vi "Main Loop.vi"(8 "error in (no error)":errorcluster, 10 "Chart Notifier":refnum<notifier>, 11 "Message Queues":T1) -> (0 "error out":errorcluster)   [LabVIEW 2018, in "Flow Module.lvlib" / "Flow Module Engine.lvlib"]
uses:
  Flow Module Engine.lvlib
  Flow Message Queues.ctl
  support/Message Queue/Message Cluster.ctl
  State Cluster.ctl
  State Enum.ctl
  Feed Module/Controls/Flow Module Settings Cluster.ctl
  Bronkhorst M13 Flow Meter/Settings Cluster.ctl
  Bronkhorst M14 Flow Meter/Settings Cluster.ctl
  Feed Module/Controls/Flow Module Display.ctl
  <vilib>/Platform/TimedLoop/XDataNode/timing_clust.ctl
  <vilib>/Platform/TimedLoop/XDataNode/nitl_modes.ctl
  <vilib>/Platform/TimedLoop/XDataNode/wakeup.ctl
  Tag VIs/Tag FGV Operation Enum.ctl
  support/Message Queue/Enqueue Message (Single).vi
  <vilib>/Platform/TimedLoop/XDataNode/XDataNode.xnode
  support/Message Queue/Message Queue.lvlib
  <vilib>/Platform/TimedLoop/XDataNode/XDNodeRunTimeDep.lvlib
  Flow Module.lvlib
  Shared Variables/Dynamic Shared Variables.lvlib
  support/Support Library.lvlib
  Bronkhorst M14 Flow Meter/Bronkhorst M14 Flow Meter.lvlib
  Bronkhorst M13 Flow Meter/Bronkhorst M13 Flow Meter.lvlib
panel:
  out "Period (s)":dbl format="%_4g"
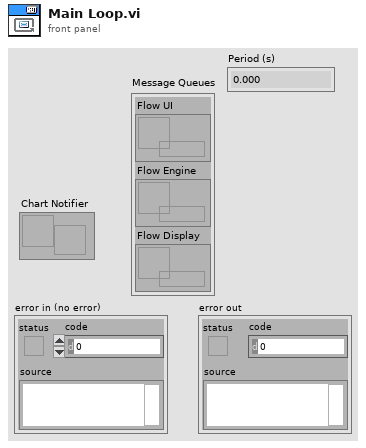
[diagram p1: front panel]
types:
  T1 = typedef "Flow Module.lvlib/Flow Message Queues.ctl" = cluster{"Flow UI":refnum<queue>, "Flow Engine":refnum<queue>, "Flow Display":refnum<queue>}
  T2 = typedef "Flow Module.lvlib/Flow Module Engine.lvlib/State Cluster.ctl" = cluster{"State":T3, "Start Time":timestamp, "Configuration":T4, "Current Time":timestamp, "First Iteration":bool, "Data":cluster{"Flow Meter Read(g/min)":dbl, "Density":dbl, "Temp (C)":dbl, "Totalized":dbl}, "Process Name":string, "Log Started":bool}
  T3 = typedef "Flow Module.lvlib/Flow Module Engine.lvlib/State Enum.ctl" = enum16{"Measuring", "Idle"}
  T4 = typedef "Flow Module.lvlib/Flow Module Settings Cluster.ctl" = cluster{"Cycle Period":dbl, "Flow Meter Type":string, "Bronkhorst M13 Settings":T5, "Bronkhorst M14 Settings":T6, "Reset Totalizer":bool}
  T5 = typedef "Bronkhorst M13 Flow Meter.lvlib/Settings Cluster.ctl" = cluster{"VISA resource name":refnum<visa-resource-name>, "Simulated?":bool, "Smoothing Steps":i32}
  T6 = typedef "Bronkhorst M14 Flow Meter.lvlib/Settings Cluster.ctl" = cluster{"VISA resource name":refnum<visa-resource-name>, "Simulated?":bool, "Smoothing Steps":i32}
  T7 = typedef "XDNodeRunTimeDep.lvlib/timing_clust.ctl" = cluster{"Expected End [f-1]":u64, "Actual End [f-1]":u64, "Finished Late? [f-1]":bool, "Expected End [i-1]":u64, "Actual End [i-1]":u64, "Finished Late? [i-1]":bool, "Expected Start [i]":u64, "Actual Start [i]":u64, "Expected Start [f]":u64, "Actual Start [f]":u64, "Source Name":string, "Structure Name":string, "Period":i64, "Deadline":i64, "Offset":i64, "Start":i64, "Priority":i32, "Timeout":i32, "Mode":T8, "Wakeup Reason":T9, "Error":errorcluster, "Source Type":string, "Secondary Source Type":string, "Global End Time":u64, "Global Start Time":u64, "Frame Duration":u64, "Iteration Duration":u64, "Assigned CPU":i32, "I/O Scan Engine Mode":u32}
  T8 = typedef "XDNodeRunTimeDep.lvlib/nitl_modes.ctl" = enum32{"No Change", "Process missed periods, maintain original phase", "Discard missed periods, maintain original phase", "Process missed periods, ignore original phase", "Discard missed periods, ignore original phase"}
  T9 = typedef "XDNodeRunTimeDep.lvlib/wakeup.ctl" = enum32{"Normal", "Aborted", "Asynchronous wakeup", "Timing source error", "Timed loop error", "Timeout"}
  T10 = cluster{"enable? (F)":bool, "name":string, "alarm on":bool, "priority":u32, "ack type":enum16{"Auto", "User", "None", "Each Occurrence"}, "area":string, "description":string, "log? (T)":bool}
  T11 = typedef "Tag FGV Operation Enum.ctl" = enum16{"Init", "Set Notification Queue", "Create Tag", "Commit", "Write Tag (Numeric)", "Write Tag (Boolean)", "Read All Tags", "Read One Tag", "Delete Tag Category", "Set Alarm Parameters (Numeric)", "Set Alarm Parameters (Boolean)", "Enable All Alarms", "Disable All Alarms", "Delete All Tags", "Read Alarms", "Ack Alarm", "Read Alarm Parameters (Numeric)", "Read Alarm Parameters (Boolean)"}
  T12 = enum32{"u32BitField", "bool", "double", "string", "int8", "uint8", "int16", "uint16", "int32", "uint32", "int64", "uint64", "single", "double waveform", "int16 waveform", "array of boolean", "array of int8", "array of uint8", "array of int16", "array of uint16", "array of int32", "array of uint32", "array of int64", "array of uint64", "array of single", "array of double", "array of double waveform", "array of int16 waveform", "array of string", "variant", "timestamp", "fixed point", "custom"}
  T13 = typedef "Flow Module.lvlib/Flow Module Display.ctl" = cluster{"Flow Value":dbl, "Cycle Period":dbl, "Density":dbl, "Temp":dbl, "Totalized":dbl}
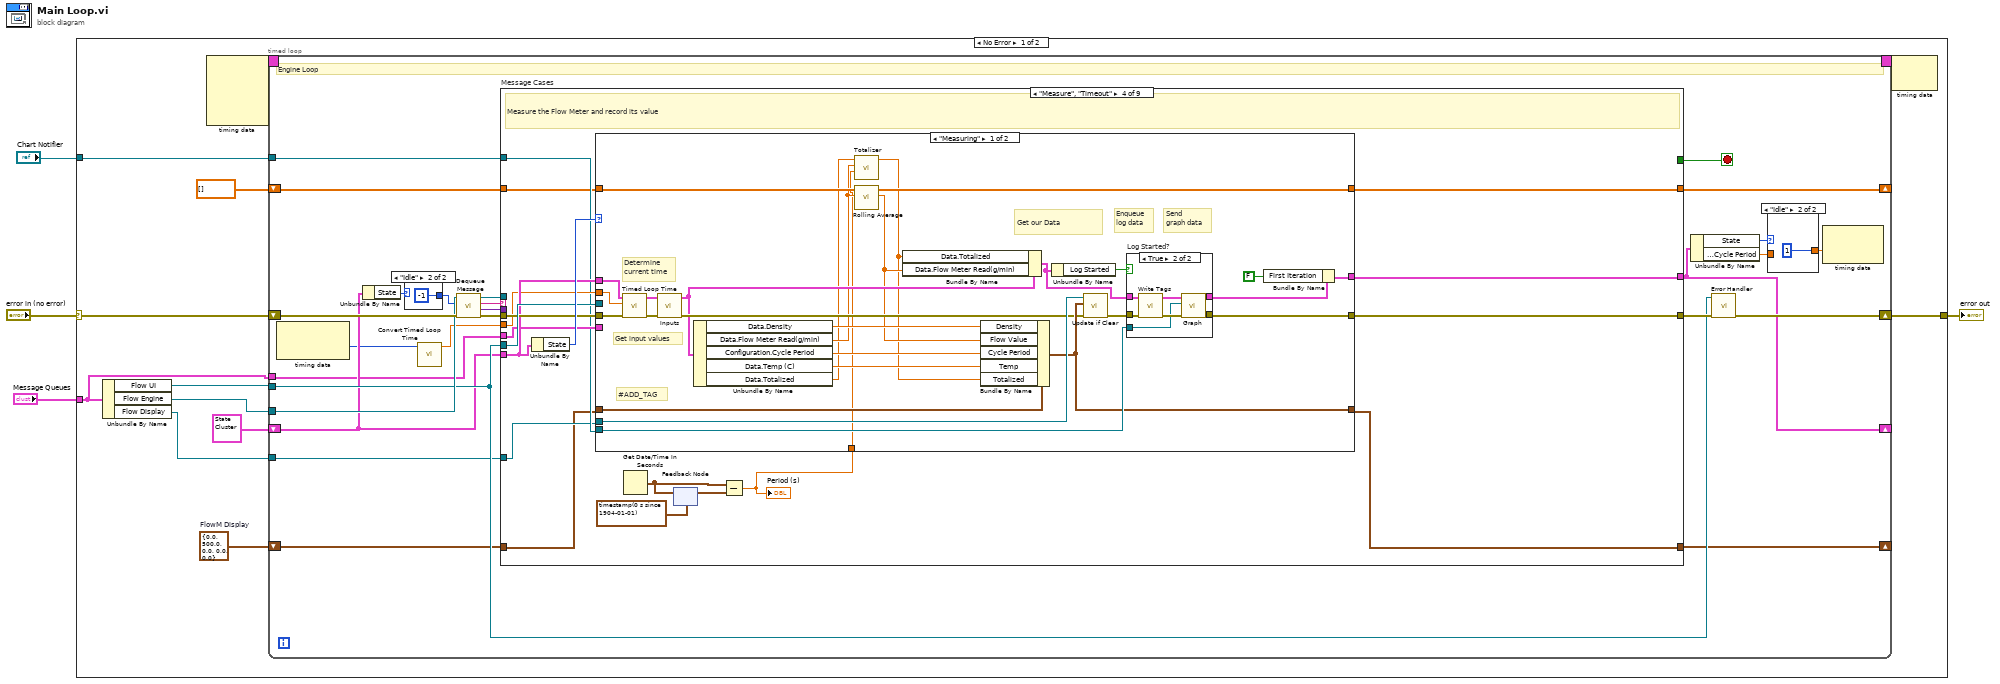
[diagram p0: block diagram]
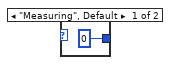
[diagram p3: hidden frame]
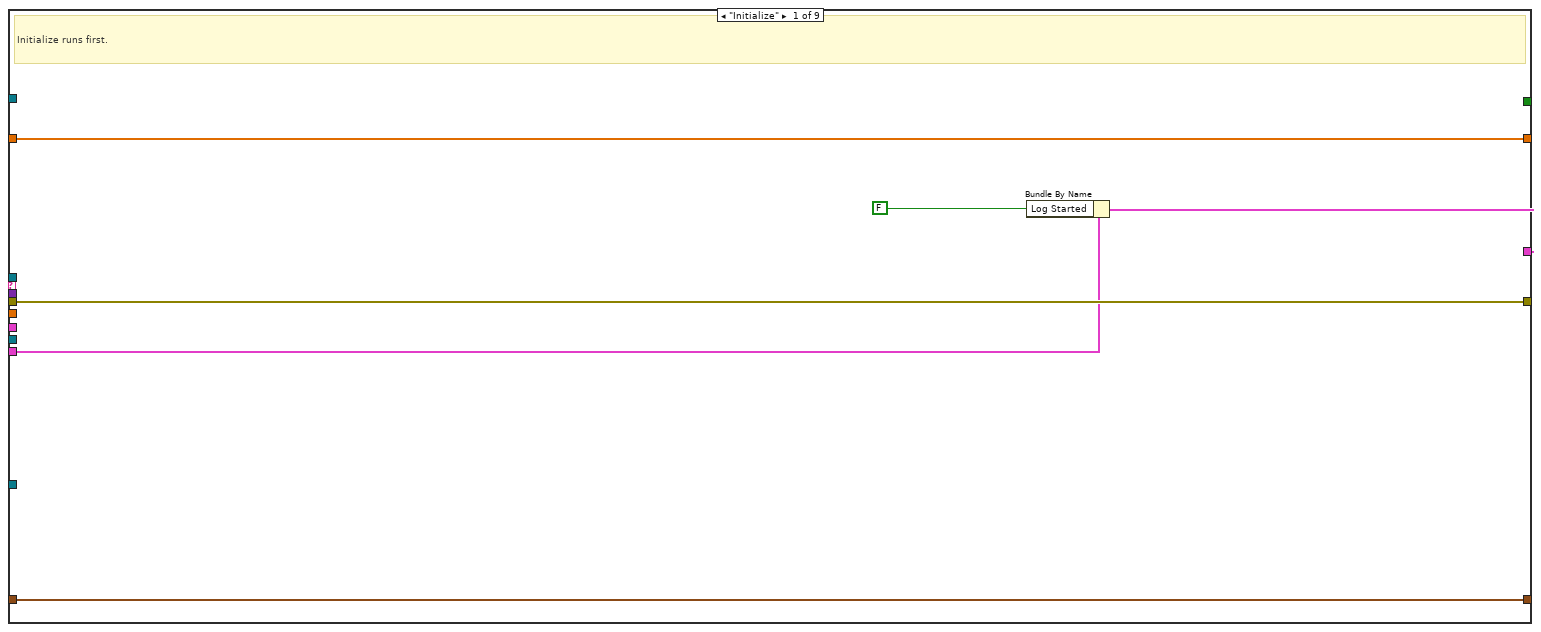
[diagram p4: hidden frame]
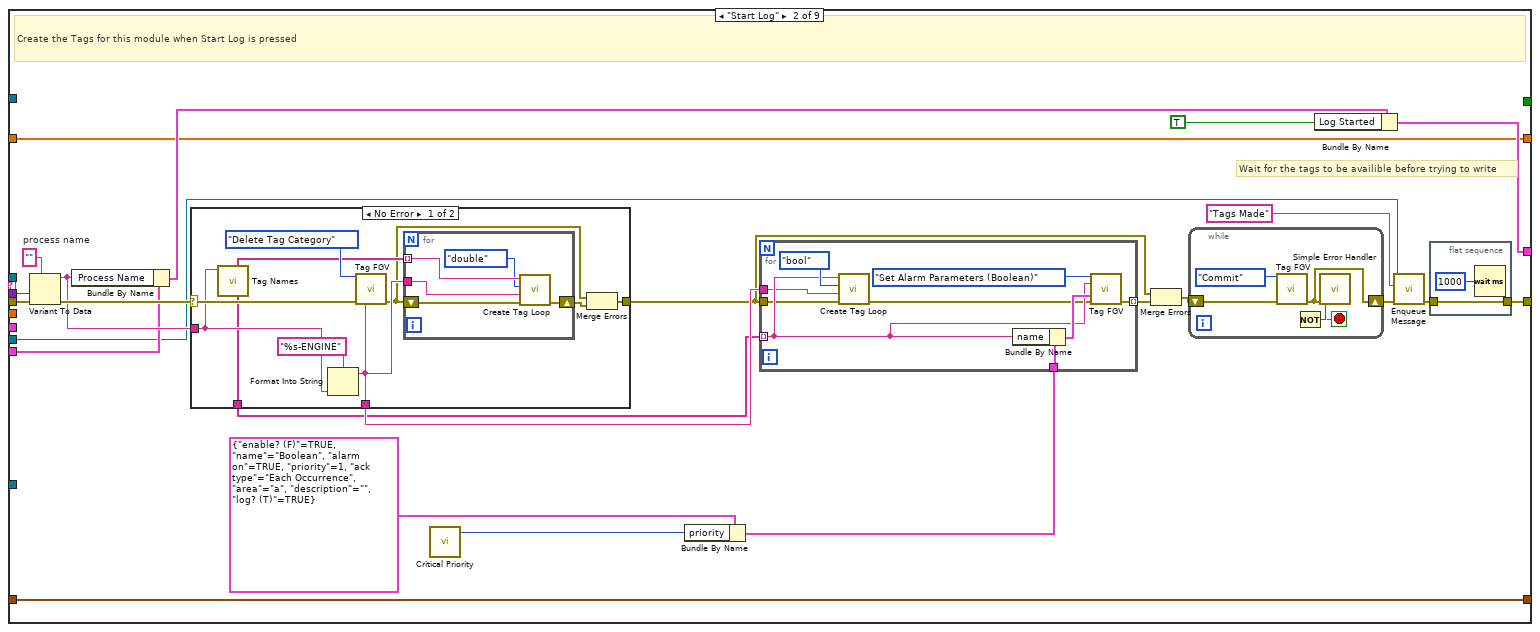
[diagram p5: hidden frame]
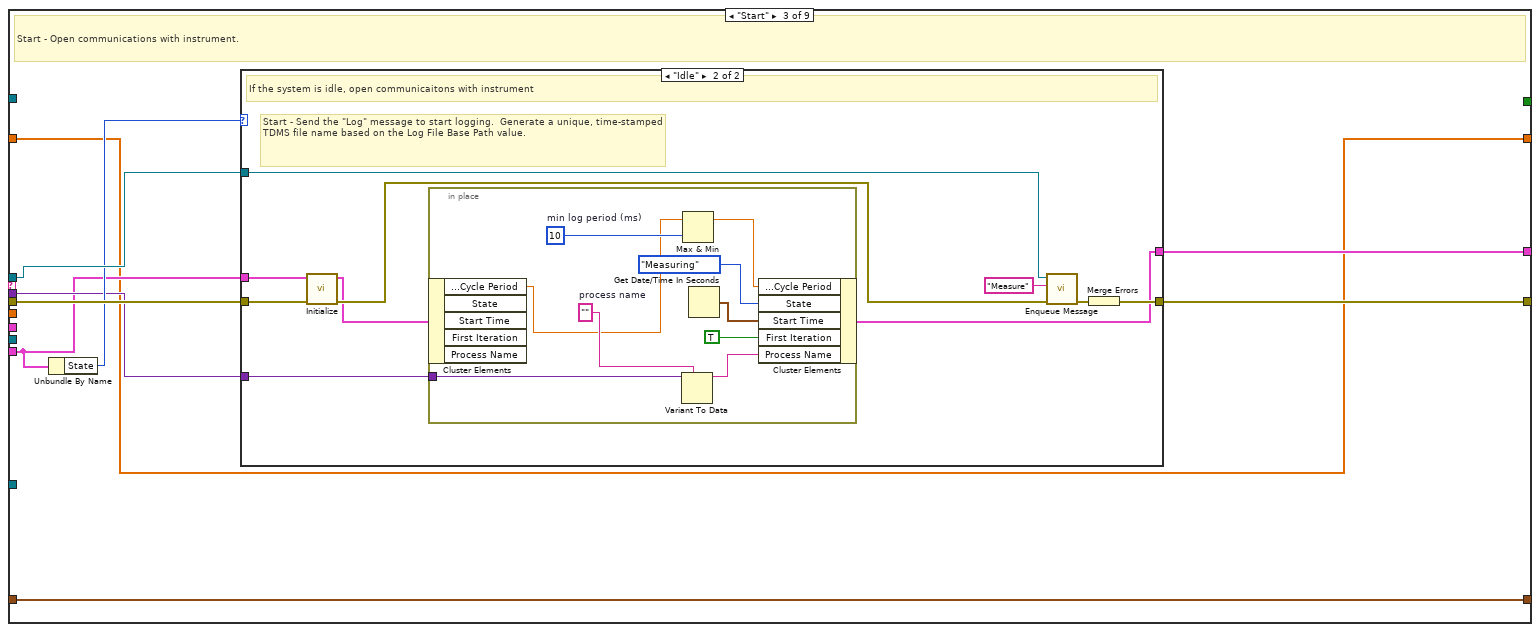
[diagram p7: hidden frame]
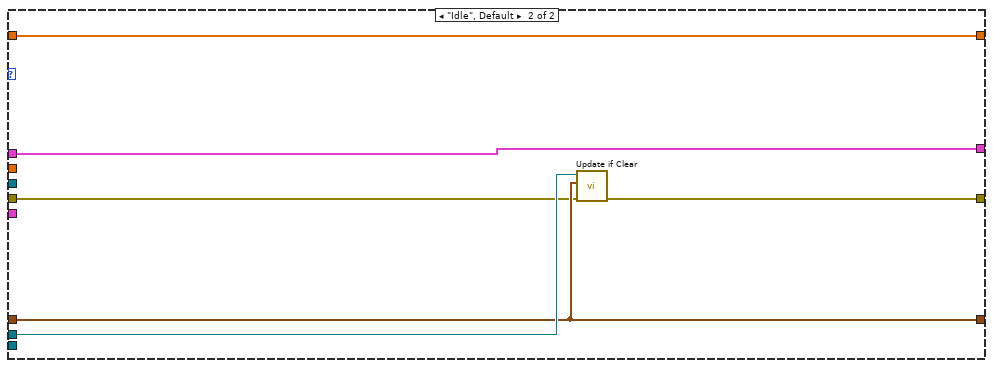
[diagram p10: hidden frame]
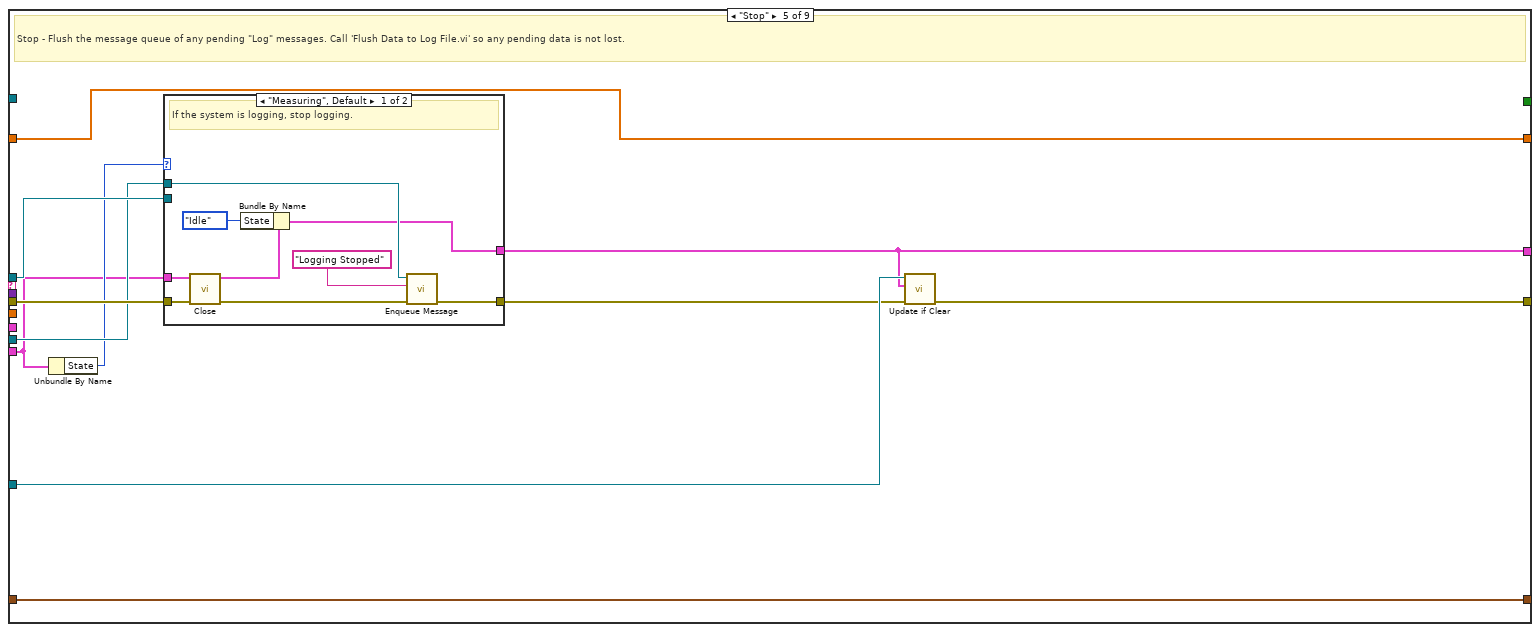
[diagram p11: hidden frame]
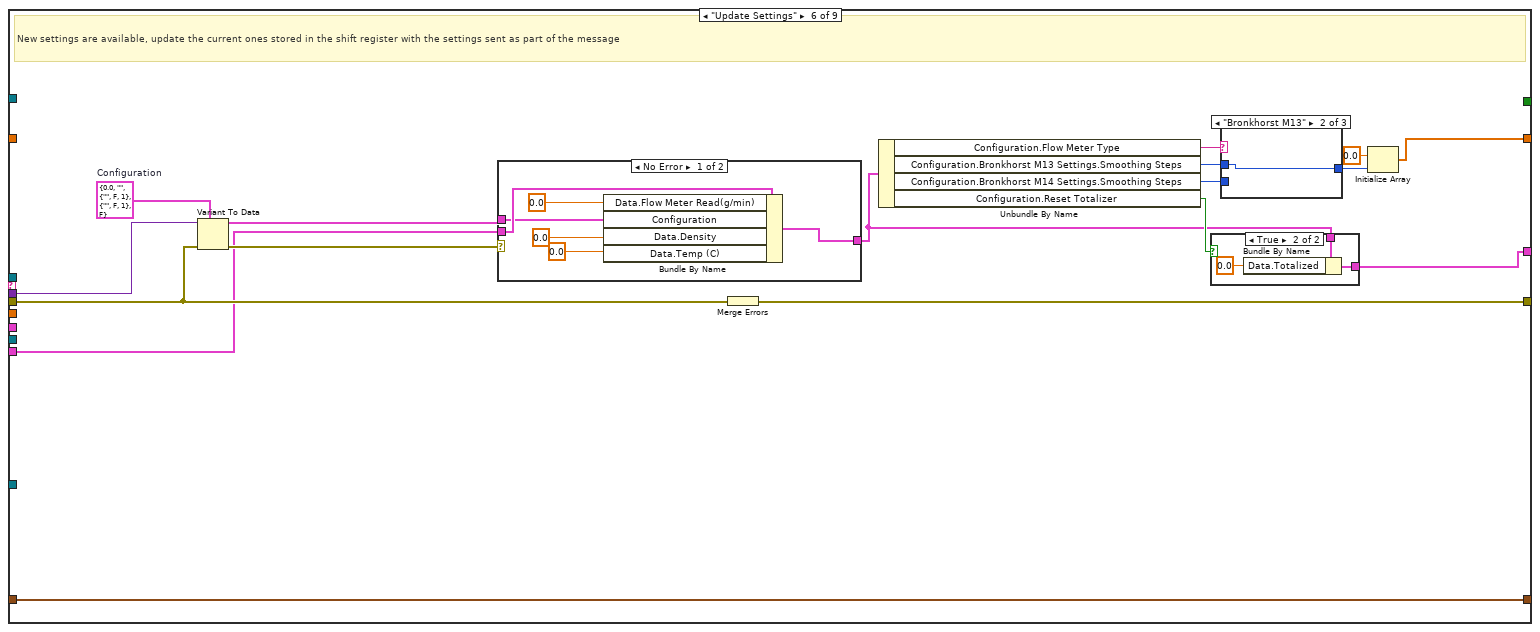
[diagram p13: hidden frame]
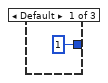
[diagram p15: hidden frame]
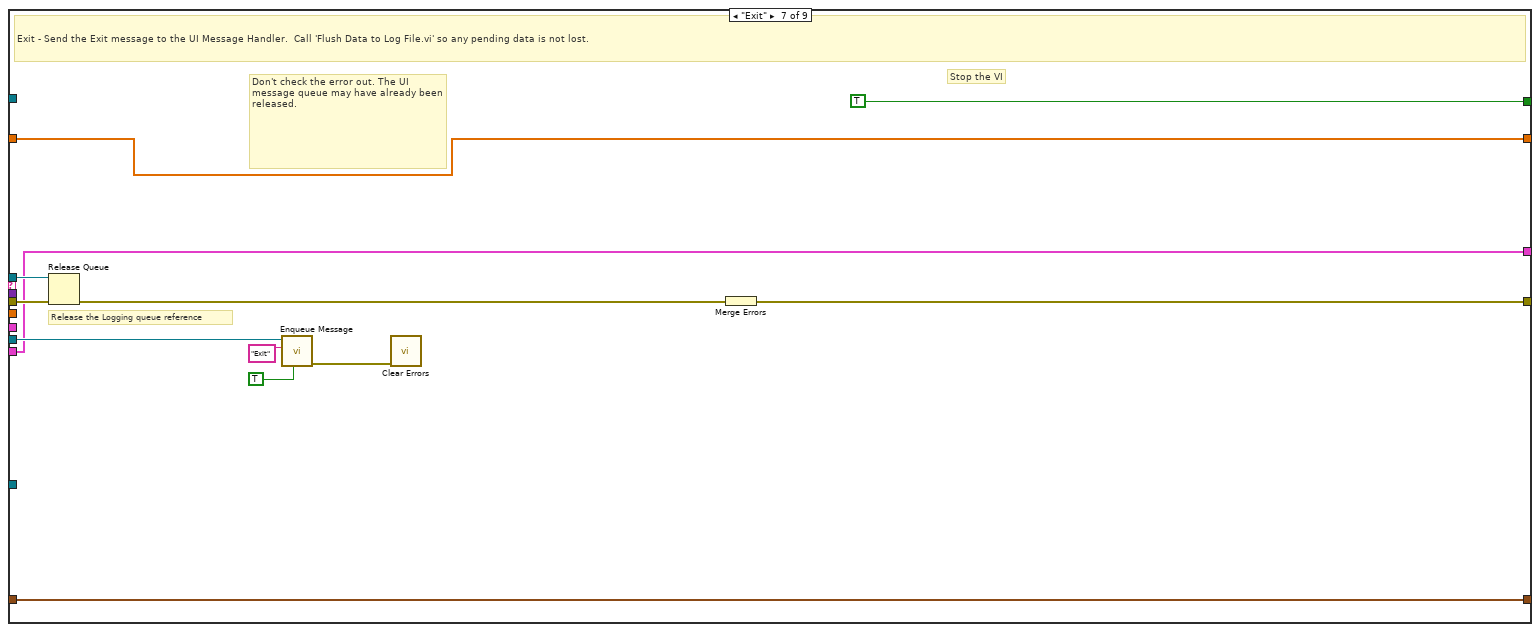
[diagram p18: hidden frame]
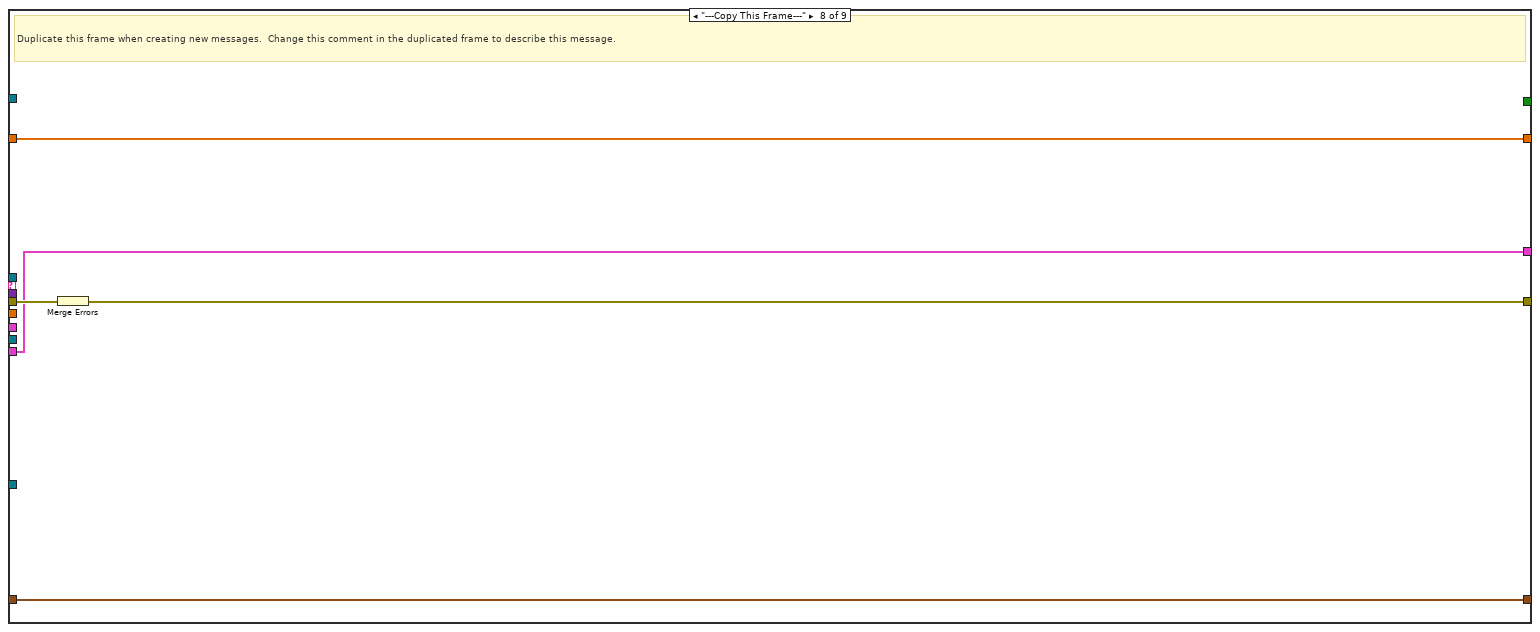
[diagram p19: hidden frame]
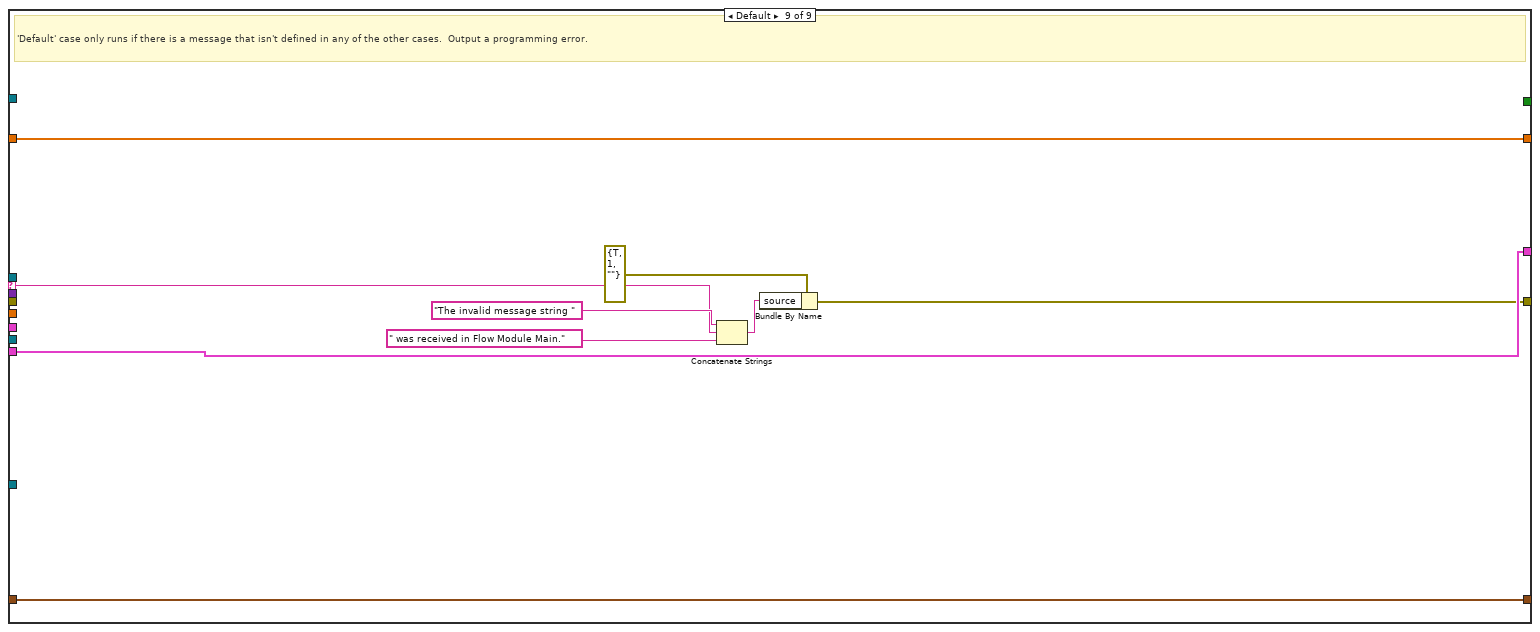
[diagram p20: hidden frame]
diagram:
  n1 = case shown="No Error" "error in (no error)" {
    selector: "error in (no error)" -> [w16 w286]
    tunnel: "Message Queues" -> [w11 _]
    tunnel: [w6 w286] -> w3
    tunnel: "Chart Notifier" -> [w9 _]
    frame No Error {
      w7 = T13 {"Flow Value"=0.0, "Cycle Period"=500.0, "Density"=0.0, "Temp"=0.0, "Totalized"=0.0}  # FlowM Display
      n2 = Unbundle By Name(w11) -> ("Flow UI"=w15:refnum<queue>, "Flow Engine"=w10:refnum<queue>, "Flow Display"=w8:refnum<queue>)
      n3 = node-c288() -> (w13:T7)  [unwired: 4 in]
      n4 = timed-loop {
        tunnel: w10 -> [w36]
        shift-right: [w20] -> _
        shift-left: T2 {"State"=enum."Idle", "Start Time"=timestamp(0 s since 1904-01-01), "Configuration"={"Cycle Period"=0.0, "Flow Meter Type"="", "Bronkhorst M13 Settings"={"VISA resource name"="", "Simulated?"=FALSE, "Smoothing Steps"=1}, "Bronkhorst M14 Settings"={"VISA resource name"="", "Simulated?"=FALSE, "Smoothing Steps"=1}, "Reset Totalizer"=FALSE}, "Current Time"=timestamp(0 s since 1904-01-01), "First Iteration"=FALSE, "Data"={"Flow Meter Read(g/min)"=0.0, "Density"=0.0, "Temp (C)"=0.0, "Totalized"=0.0}, "Process Name"="", "Log Started"=FALSE} -> [w32]
        shift-right: [w34] -> w6
        shift-left: w16 -> [w41]
        tunnel: w15 -> [w33]
        timing: w13 -> [_]
        timing-out: [_] -> w12
        tunnel: w11 -> [w24]
        tunnel: w9 -> [w23]
        tunnel: w8 -> [w22]
        shift-right: [w21] -> _
        shift-left: w7 -> [w19]
        shift-right: [w17] -> _
        shift-left: dbl[] [] -> [w18]
        stop <- w42 stop-if-true
        # "Engine Loop"
        n5 = node-c288() -> (w26:i64)  [unwired: 1 in, 1 out]
        n6 = Unbundle By Name(w32) -> ("State"=w31:T3)
        n7 = case shown="\"Idle\"" w31 {
          tunnel: [0 ("timeout in ms (-1)") -1 ("timeout in ms (-1)")] -> w30
          frame "Measuring", Default {
          }
          frame "Idle" {
          }
        }
        n8 = call "Convert Timed Loop Time.vi"("Actual Start [i]"=w26) -> ("ET since start (s)"=w25:dbl)  [unwired: 10 in]
        n9 = call "Dequeue Message.vi"("error in (no error)"=w41, "timeout in ms (-1)"=w30, "Message Queue"=w36) -> ("error out"=w40:errorcluster, "Message Data"=w38:variant, "Message"=w39:string, "dup Message Queue"=w37:refnum<queue>)  [unwired: 5 in]
        n10 = case "Message Cases" shown="\"Measure\", \"Timeout\"" w39 {
          selector: w39 -> [_ _ _ _ _ _ _ _ w277]
          tunnel: w37 -> [_ _ w121 _ w214 _ w263 _ _]
          tunnel: w40 -> [w57 w77 w120 w158 w215 w241 w266 w274 _]
          tunnel: [w57 w61 w122 w159 w206 w243 w268 w273 w276] -> w35
          tunnel: w32 -> [w55 w76 w117 w157 w211 w239 w259 w271 w282]
          tunnel: [_ _ _ _ _ _ TRUE _ _] -> w42
          tunnel: w38 -> [_ w75 w118 _ _ w242 _ _ _]
          tunnel: w33 -> [_ w64 _ w160 w213 _ w267 _ _]
          tunnel: w25 -> [_ _ _ w156 _ _ _ _ _]
          tunnel: w24 -> [_ _ _ w155 _ _ _ _ _]
          tunnel: w23 -> [_ _ _ w152 _ _ _ _ _]
          tunnel: w22 -> [_ _ _ w151 w209 _ _ _ _]
          tunnel: w19 -> [w56 w81 w116 w150 w210 w236 w260 w272 w283]
          tunnel: [w56 w81 w116 w149 w210 w236 w260 w272 w283] -> w21
          tunnel: [w54 w67 w115 w148 w208 w227 w259 w271 w282] -> w20
          tunnel: w18 -> [w52 w58 w114 w146 w205 _ w258 w270 w275]
          tunnel: [w52 w58 w114 w145 w205 w230 w258 w270 w275] -> w17
          frame "Initialize" {
            # "Initialize runs first."
            n11 = Bundle By Name(cluster=w55, "Log Started"=FALSE) -> (w54:T2)
          }
          frame "Start Log" {
            w80 = ""  # process name
            # "Wait for the tags to be availible before trying to write"
            # "Create the Tags for this module when Start Log is pressed"
            n12 = Variant To Data(error in=w77, type=w80, Variant=w75) -> (data=w78:string, error out=w79:errorcluster)
            n13 = Bundle By Name(cluster=w76, "Process Name"=w78) -> (w68:T2)
            n14 = case shown="No Error" w79 {
              selector: w79 -> [w105 w113]
              tunnel: [w99 w113] -> w59
              tunnel: w78 -> [w104 _]
              tunnel: [w102 _] -> w74
              tunnel: [w101 _] -> w73
              frame No Error {
                n15 = call "Tag Names.vi"("Process Name"=w104) -> ("All Boolean Tags"=w101:string[], "All  Numeric Tags"=w103:string[])  [unwired: 8 in, 1 out]
                n16 = Format Into String(format string="%s-ENGINE", w104) -> (resulting string=w102:string)  [unwired: 2 in, 1 out]
                n17 = call "Tag FGV.vi"("Operation"=Tag_FGV_Operation_Enum."Delete Tag Category", "error in (no error)"=w105, "Tag Category"=w102) -> ("error out"=w98:errorcluster)  [unwired: 5 in, 7 out]
                n18 = for {
                  shift-right: [w108] -> w100
                  shift-left: w98 -> [w109]
                  tunnel: w102 -> [w111]
                  tunnel: w103 -> [w112] mode=indexing
                  n19 = call "Create Tag Loop.vi"("error in (no error)"=w109, "Tag Category"=w111, "data type"=T12."double", "Tag Name"=w112) -> ("error out"=w108:errorcluster)  [unwired: 7 in]
                }
                n20 = Merge Errors(w98, w100) -> (w99:errorcluster)
              }
              frame Error {
              }
            }
            n21 = call "Critical Priority.vi"() -> ("critical priority"=w70:i32)  [unwired: 11 in]
            n22 = Bundle By Name(cluster=T10 {"enable? (F)"=TRUE, "name"="Boolean", "alarm on"=TRUE, "priority"=1, "ack type"=enum."Each Occurrence", "area"="a", "description"="", "log? (T)"=TRUE} ("Boolean alarm settings"), "priority"=w70) -> (w69:T10)
            n23 = for {
              tunnel: w69 -> [w97]
              tunnel: [w96] -> w72 mode=indexing
              tunnel: w73 -> [w92] mode=indexing
              tunnel: w59 -> [w90]
              tunnel: w74 -> [w91]
              n24 = call "Create Tag Loop.vi"("error in (no error)"=w90, "Tag Category"=w91, "data type"=T12."bool", "Tag Name"=w92) -> ("error out"=w89:errorcluster)  [unwired: 7 in]
              n25 = Bundle By Name(cluster=w97, "name"=w92) -> (w95:T10)
              n26 = call "Tag FGV.vi"("Operation"=Tag_FGV_Operation_Enum."Set Alarm Parameters (Boolean)", "Tag Name"=w92, "Data"=w95, "error in (no error)"=w89) -> ("error out"=w96:errorcluster)  [unwired: 4 in, 7 out]
            }
            n27 = Merge Errors(w59, w72) -> (w63:errorcluster)
            n28 = while {
              shift-right: [w86] -> w62
              shift-left: w63 -> [w87]
              stop <- w84 stop-if-true
              n29 = call "Tag FGV.vi"("Operation"=Tag_FGV_Operation_Enum."Commit", "error in (no error)"=w87) -> ("error out"=w86:errorcluster)  [unwired: 6 in, 7 out]
              n30 = call <vilib>:"Simple Error Handler.vi"("error in (no error)"=w86) -> ("error?"=w85:bool)  [unwired: 4 in, 4 out]
              n31 = Not(x=w85) -> (.not. x?=w84:bool)
            }
            n32 = Bundle By Name(cluster=w68, "Log Started"=TRUE) -> (w67:T2)
            n33 = call-poly "Enqueue Message.vi"("error in (no error)"=w62, "Message"="Tags Made", "Message Queue"=w64) -> ("error out"=w60:errorcluster)  [unwired: 7 in, 1 out]
            n34 = flat-sequence {
              tunnel: [w82] -> w61
              tunnel: w60 -> [w82]
              frame #0 {
                n35 = Wait (ms)(milliseconds to wait=u32 1000) -> ()  [unwired: 1 out]
              }
            }
          }
          frame "Start" {
            # "Start - Open communications with instrument."
            n36 = Unbundle By Name(w117) -> ("State"=w119:T3)
            n37 = case shown="\"Idle\"" w119 {
              tunnel: [w123 w134] -> w122
              tunnel: w121 -> [_ w131]
              tunnel: w120 -> [w123 w129]
              tunnel: w117 -> [w124 w128]
              tunnel: [w124 w125] -> w115
              tunnel: w118 -> [_ w127]
              frame "Measuring", Default {
                # "The system is already running. Ignore the \"Start\" message."
              }
              frame "Idle" {
                # "Start - Send the \"Log\" message to start logging.  Generate a unique, time-stamped TDMS file name based on the Log File Base Path value."
                # "If the system is idle, open communicaitons with instrument"
                n38 = call "Initialize.vi"("error in (no error)"=w129, "State in"=w128) -> ("error out"=w130:errorcluster, "State out"=w126:T2)  [unwired: 8 in]
                n39 = in-place {
                  in-place-border: w127 -> [w141]
                  w142 = ""  # process name
                  w143 = 10  # min log period (ms)
                  n40 = in-place-cluster #1(w126) -> ("Configuration.Cycle Period"=w135:dbl)  [unwired: 4 out]
                  n41 = Variant To Data(type=w142, Variant=w141) -> (data=w136:string)  [unwired: 1 in, 1 out]
                  n42 = Max & Min(x=w135, y=w143) -> (max(x,y)=w140:dbl)  [unwired: 1 out]
                  n43 = Get Date/Time In Seconds() -> (seconds since 1Jan1904=w138:timestamp)
                  n44 = in-place-cluster #1("Configuration.Cycle Period"=w140, "State"=State_Enum."Measuring", "Start Time"=w138, "First Iteration"=TRUE, "Process Name"=w136) -> (w125:T2)
                }
                n45 = call-poly "Enqueue Message.vi"("error in (no error)"=w130, "Message"="Measure", "Message Queue"=w131) -> ("error out"=w132:errorcluster)  [unwired: 7 in, 1 out]
                n46 = Merge Errors(w132) -> (w134:errorcluster)
              }
            }
          }
          frame "Measure", "Timeout" {
            # "Measure the Flow Meter and record its value"
            n47 = Unbundle By Name(w157) -> ("State"=w161:T3)
            n48 = Get Date/Time In Seconds() -> (seconds since 1Jan1904=w153:timestamp)
            n49 = feedback-in #2(w153) -> ()
            n50 = feedback #2(timestamp(0 s since 1904-01-01) ("seconds since 1Jan1904")) -> (w154:timestamp)
            n51 = Subtract(x=w153, y=w154) -> (x-y=w144:dbl)
            "Period (s)" <- w144
            n52 = case shown="\"Measuring\"" w161 {
              tunnel: w158 -> [w187 w201]
              tunnel: w157 -> [w185 w204]
              tunnel: w160 -> [_ _]
              tunnel: [w189 w200] -> w159
              tunnel: [w182 w204] -> w148
              tunnel: w156 -> [w184 _]
              tunnel: w155 -> [_ _]
              tunnel: w152 -> [w180 _]
              tunnel: w151 -> [w174 w203]
              tunnel: w150 -> [w179 w202]
              tunnel: [w173 w202] -> w149
              tunnel: w146 -> [w170 w199]
              tunnel: [w169 w199] -> w145
              tunnel: w144 -> [w164 _]
              frame "Measuring" {
                # "Get our Data"
                # "#ADD_TAG"
                # "Determine\ncurrent time"
                # "Send\ngraph data"
                # "Enqueue\nlog data"
                # "Get input values"
                n53 = call "Timed Loop Time.vi"("error in (no error)"=w187, "ET since start (s)"=w184, "State in"=w185) -> ("error out"=w188:errorcluster, "State out"=w186:T2)  [unwired: 7 in]
                n54 = call "Inputs.vi"("error in (no error)"=w188, "State in"=w186) -> ("error out"=w172:errorcluster, "State out"=w168:T2)  [unwired: 8 in]
                n55 = Unbundle By Name(w168) -> ("Data.Density"=w177:dbl, "Data.Flow Meter Read(g/min)"=w165:dbl, "Configuration.Cycle Period"=w178:dbl, "Data.Temp (C)"=w176:dbl, "Data.Totalized"=w163:dbl)
                n56 = call "Totalizer.vi"("Period"=w164, "Flow Rate"=w165, "Current Total"=w163) -> ("New Total"=w162:dbl)  [unwired: 8 in]
                n57 = call "Rolling Average.vi"("New Value"=w165, "Old Array"=w170) -> ("Calculated Value"=w167:dbl, "New Array"=w169:dbl[])  [unwired: 8 in]
                n58 = Bundle By Name(cluster=w168, "Data.Totalized"=w162, "Data.Flow Meter Read(g/min)"=w167) -> (w166:T2)
                n59 = Bundle By Name(cluster=w179, "Density"=w177, "Flow Value"=w167, "Cycle Period"=w178, "Temp"=w176, "Totalized"=w162) -> (w173:T13)
                n60 = Unbundle By Name(w166) -> ("Log Started"=w175:bool)
                n61 = call "Update if Clear.vi"("error in (no error)"=w172, "Message Data"=w173, "Queue in"=w174) -> ("error out"=w171:errorcluster)  [unwired: 8 in]
                n62 = case "Log Started?" shown="True" w175 {
                  tunnel: [w191 w196] -> w189
                  tunnel: [w190 w195] -> w183
                  tunnel: w180 -> [_ w194]
                  tunnel: w171 -> [w191 w193]
                  tunnel: w166 -> [w190 w192]
                  frame False {
                  }
                  frame True {
                    n63 = call "Write Tags.vi"("error in (no error)"=w193, "State in"=w192) -> ("error out"=w197:errorcluster, "State out"=w198:T2)  [unwired: 8 in]
                    n64 = call "Graph.vi"("error in (no error)"=w197, "notifier out"=w194, "State in"=w198) -> ("error out"=w196:errorcluster, "State out"=w195:T2)  [unwired: 7 in]
                  }
                }
                n65 = Bundle By Name(cluster=w183, "First Iteration"=FALSE) -> (w182:T2)
              }
              frame "Idle", Default {
                n66 = call "Update if Clear.vi"("error in (no error)"=w201, "Message Data"=w202, "Queue in"=w203) -> ("error out"=w200:errorcluster)  [unwired: 8 in]
              }
            }
          }
          frame "Stop" {
            # "Stop - Flush the message queue of any pending \"Log\" messages. Call 'Flush Data to Log File.vi' so any pending data is not lost."
            n67 = Unbundle By Name(w211) -> ("State"=w212:T3)
            n68 = case shown="\"Measuring\", Default" w212 {
              tunnel: [w220 w226] -> w207
              tunnel: w215 -> [w217 w226]
              tunnel: w214 -> [_ _]
              tunnel: w213 -> [w224 _]
              tunnel: w211 -> [w218 w225]
              tunnel: [w222 w225] -> w208
              frame "Measuring", Default {
                # "If the system is logging, stop logging."
                n69 = call "Close.vi"("error in (no error)"=w217, "State in"=w218) -> ("error out"=w216:errorcluster, "State out"=w219:T2)  [unwired: 8 in]
                n70 = Bundle By Name(cluster=w219, "State"=State_Enum."Idle") -> (w222:T2)
                n71 = call-poly "Enqueue Message.vi"("error in (no error)"=w216, "Message"="Logging Stopped", "Message Queue"=w224) -> ("error out"=w220:errorcluster)  [unwired: 7 in, 1 out]
              }
              frame "Idle" {
                # "The system is already idle. Ignore the \"Stop\" message."
              }
            }
            n72 = call "Update if Clear.vi"("error in (no error)"=w207, "Message Data"=w208, "Queue in"=w209) -> ("error out"=w206:errorcluster)  [unwired: 8 in]
          }
          frame "Update Settings" {
            w237 = T4 {"Cycle Period"=0.0, "Flow Meter Type"="", "Bronkhorst M13 Settings"={"VISA resource name"="", "Simulated?"=FALSE, "Smoothing Steps"=1}, "Bronkhorst M14 Settings"={"VISA resource name"="", "Simulated?"=FALSE, "Smoothing Steps"=1}, "Reset Totalizer"=FALSE}  # Configuration
            # "New settings are available, update the current ones stored in the shift register with the settings sent as part of the message"
            n73 = Variant To Data(error in=w241, type=w237, Variant=w242) -> (data=w238:T4, error out=w240:errorcluster)
            n74 = case shown="No Error" w240 {
              tunnel: w239 -> [w256 w257]
              tunnel: w238 -> [w255 _]
              tunnel: [w254 w257] -> w228
              frame No Error {
                n75 = Bundle By Name(cluster=w256, "Data.Flow Meter Read(g/min)"=0.0 ("Data.Scale Read(g)"), "Configuration"=w255, "Data.Density"=0.0, "Data.Temp (C)"=0.0 ("Data.Density")) -> (w254:T2)
              }
              frame Error {
              }
            }
            n76 = Merge Errors(w241) -> (w243:errorcluster)
            n77 = Unbundle By Name(w228) -> ("Configuration.Flow Meter Type"=w235:string, "Configuration.Bronkhorst M13 Settings.Smoothing Steps"=w234:i32, "Configuration.Bronkhorst M14 Settings.Smoothing Steps"=w233:i32, "Configuration.Reset Totalizer"=w229:bool)
            n78 = case shown="True" w229 {
              tunnel: w228 -> [w244 w247]
              tunnel: [w244 w245] -> w227
              frame False {
              }
              frame True {
                n79 = Bundle By Name(cluster=w247, "Data.Totalized"=0.0) -> (w245:T2)
              }
            }
            n80 = case shown="\"Bronkhorst M13\"" w235 {
              tunnel: w234 -> [_ w249 _]
              tunnel: w233 -> [_ _ w250]
              tunnel: [1 ("Smoothing Steps") w249 w250] -> w232
              frame Default {
              }
              frame "Bronkhorst M13" {
              }
              frame "Bronkhorst M14" {
              }
            }
            n81 = Initialize Array(0.0 ("element"), w232) -> (w230:dbl[])
          }
          frame "Exit" {
            # "Release the Logging queue reference"
            # "Don't check the error out. The UI message queue may have already been released."
            # "Stop the VI"
            # "Exit - Send the Exit message to the UI Message Handler.  Call 'Flush Data to Log File.vi' so any pending data is not lost."
            n82 = Release Queue(queue=w263, error in (no error)=w266) -> (error out=w262:errorcluster)  [unwired: 1 in, 2 out]
            n83 = call-poly "Enqueue Message.vi"("Priority Message? (F)"=TRUE, "Message"="Exit", "Message Queue"=w267) -> ("error out"=w261:errorcluster)  [unwired: 7 in, 1 out]
            n84 = call <vilib>:"Clear Errors.vi"("error in (no error)"=w261) -> ()  [unwired: 5 in, 2 out]
            n85 = Merge Errors(w262) -> (w268:errorcluster)
          }
          frame "---Copy This Frame---" {
            # "Duplicate this frame when creating new messages.  Change this comment in the duplicated frame to describe this message."
            n86 = Merge Errors(w274) -> (w273:errorcluster)
          }
          frame Default {
            # "'Default' case only runs if there is a message that isn't defined in any of the other cases.  Output a programming error."
            n87 = Concatenate Strings("The invalid message string " ("string"), w277, " was received in Flow Module Main." ("string")) -> (w278:string)
            n88 = Bundle By Name(cluster=errorcluster {"status"=TRUE, "code"=1, "source"=""} ("error constant"), "source"=w278) -> (w276:errorcluster)
          }
        }
        n89 = Unbundle By Name(w20) -> ("State"=w29:T3, "Configuration.Cycle Period"=w27:dbl)
        n90 = call "Error Handler.vi"("error in (no error)"=w35, "Message Queue"=w33) -> ("dup error in"=w34:errorcluster)  [unwired: 8 in, 1 out]
        n91 = case shown="\"Idle\"" w29 {
          tunnel: [w43 1] -> w28
          tunnel: w27 -> [w43 _]
          frame "Measuring" {
          }
          frame "Idle" {
          }
        }
        n92 = node-c288(w28) -> ()  [unwired: 1 in, 1 out]
      }
      n93 = node-c288(w12) -> ()  [unwired: 1 out]
    }
    frame Error {
    }
  }
  "error out" <- w3
